vi "Update Coin Reserve.vi"(7 "Add/Sub":T2, 8 "error in (no error)":errorcluster, 9 "Currency In":T3, 10 "Data In":T4, 11 "Coin":T1) -> (0 "error out":errorcluster, 1 "Currency Out":T3, 2 "Data out":T4)   [LabVIEW 2026]
uses:
  controls/Data.ctl
  controls/Currency.ctl
  controls/Currency Enum.ctl
  controls/Coin Reserve Enum.ctl
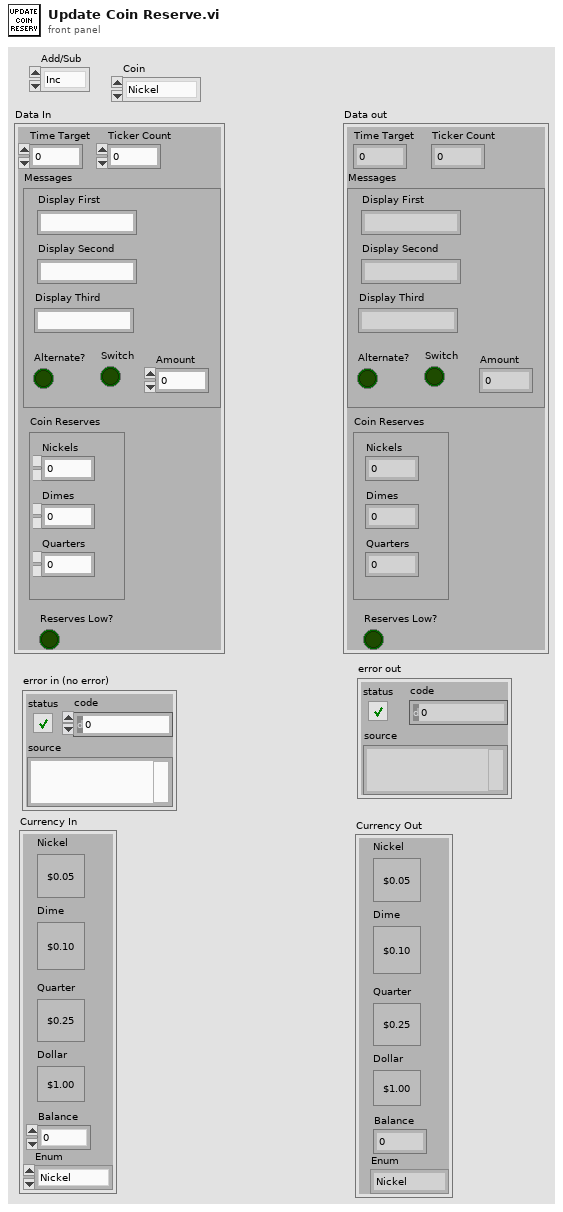
[diagram p1: front panel]
types:
  T1 = typedef "Currency Enum.ctl" = enum16{"Nickel", "Dime", "Quarter", "Dollar"}
  T2 = typedef "Coin Reserve Enum.ctl" = enum16{"Inc", "Dec"}
  T3 = typedef "Currency.ctl" = cluster{"Nickel":bool, "Dime":bool, "Quarter":bool, "Dollar":bool, "Balance":dbl, "Enum":T1}
  T4 = typedef "Data.ctl" = cluster{"Time Target":dbl, "Messages":cluster{"Display First":string, "Display Second":string, "Alternate?":bool, "Switch":bool, "Display Third":string, "Amount":i32}, "Ticker Count":dbl, "Coin Reserves":cluster{"Nickels":i32, "Dimes":i32, "Quarters":i32}, "Reserves Low?":bool}
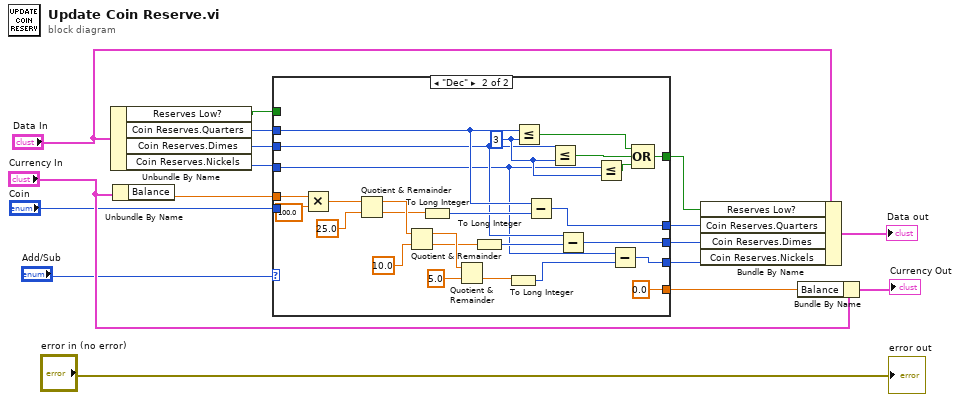
[diagram p0: block diagram]
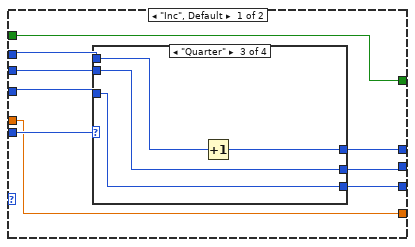
[diagram p2: hidden frame]
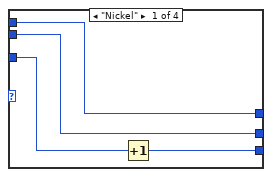
[diagram p3: hidden frame]
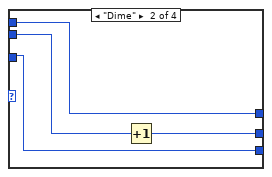
[diagram p4: hidden frame]
diagram:
  n1 = Unbundle By Name("Data In") -> ("Reserves Low?"=w3:bool, "Coin Reserves.Quarters"=w16:i32, "Coin Reserves.Dimes"=w11:i32, "Coin Reserves.Nickels"=w8:i32)
  n2 = Unbundle By Name("Currency In") -> ("Balance"=w7:dbl)
  n3 = case shown="\"Dec\"" "Add/Sub" {
    tunnel: w16 -> [w20 w52]
    tunnel: [w19 w51] -> w15
    tunnel: [w25 w50] -> w13
    tunnel: w11 -> [w22 w49]
    tunnel: [w21 w47] -> w10
    tunnel: [w23 w45] -> w9
    tunnel: w8 -> [w24 w44]
    tunnel: w7 -> [w18 w43]
    tunnel: "Coin" -> [w26 _]
    tunnel: w3 -> [w25 _]
    tunnel: [w18 0.0 ("Balance")] -> w1
    frame "Inc", Default {
      n4 = case shown="\"Quarter\"" w26 {
        tunnel: w24 -> [w30 w31 w36 w41]
        tunnel: [w29 w31 w36 w41] -> w23
        tunnel: w22 -> [w27 w34 w35 w40]
        tunnel: [w27 w33 w35 w40] -> w21
        tunnel: w20 -> [w28 w32 w38 w39]
        tunnel: [w28 w32 w37 w39] -> w19
        frame "Nickel" {
          n5 = Increment(x=w30) -> (x+1=w29:i32)
        }
        frame "Dime" {
          n6 = Increment(x=w34) -> (x+1=w33:i32)
        }
        frame "Quarter" {
          n7 = Increment(x=w38) -> (x+1=w37:i32)
        }
        frame Default {
        }
      }
    }
    frame "Dec" {
      w60 = 3 ("y")
      n8 = Multiply(x=w43, y=100.0) -> (x*y=w63:dbl)
      n9 = Quotient & Remainder(x=w63, y=25.0) -> (x-y*floor(x/y)=w62:dbl, floor(x/y)=w56:dbl)
      n10 = Quotient & Remainder(x=w62, y=10.0) -> (x-y*floor(x/y)=w61:dbl, floor(x/y)=w55:dbl)
      n11 = To Long Integer(number=w56) -> (32bit integer=w53:i32)
      n12 = Quotient & Remainder(x=w61, y=5.0) -> (floor(x/y)=w54:dbl)  [unwired: 1 out]
      n13 = To Long Integer(number=w55) -> (32bit integer=w48:i32)
      n14 = To Long Integer(number=w54) -> (32bit integer=w46:i32)
      n15 = Less Or Equal?(x=w52, y=w60) -> (x <= y?=w59:bool)
      n16 = Subtract(x=w52, y=w53) -> (x-y=w51:i32)
      n17 = Less Or Equal?(x=w49, y=w60) -> (x <= y?=w58:bool)
      n18 = Subtract(x=w49, y=w48) -> (x-y=w47:i32)
      n19 = Less Or Equal?(x=w44, y=w60) -> (x <= y?=w57:bool)
      n20 = Subtract(x=w44, y=w46) -> (x-y=w45:i32)
      n21 = Compound Arithmetic op=OR(w59, w58, w57) -> (w50:bool)
    }
  }
  n22 = Bundle By Name(cluster="Data In", "Reserves Low?"=w13, "Coin Reserves.Quarters"=w15, "Coin Reserves.Dimes"=w10, "Coin Reserves.Nickels"=w9) -> (→"Data out":T4)
  n23 = Bundle By Name(cluster="Currency In", "Balance"=w1) -> (→"Currency Out":T3)
  "error out" <- "error in (no error)"
